vi "Kto_był_pierwszy_SUBVI.vi"(6 "Brama 2":T2, 7 "Brama 1":T2, 9 "Wejscie":T1) -> (3 "output cluster":T1)   [LabVIEW 2017]
panel:
  in  "Cluster":T1
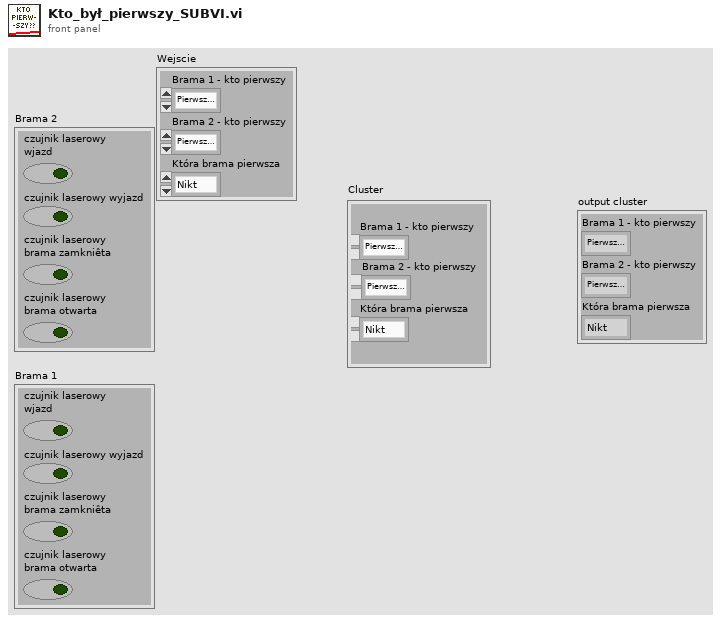
[diagram p1: front panel]
types:
  T1 = cluster{"Brama 1 - kto pierwszy":enum16{"Pierwszy wjazd", "Nikt", "Pierwszy wyjazd"}, "Brama 2 - kto pierwszy":enum16{"Pierwszy wjazd", "Nikt", "Pierwszy wyjazd"}, "Która brama pierwsza":enum16{"Nikt", "Brama 1", "Brama 2"}}
  T2 = cluster{"czujnik laserowy \nwjazd":bool, "czujnik laserowy wyjazd":bool, "czujnik laserowy \nbrama zamkniêta":bool, "czujnik laserowy \nbrama otwarta":bool}
  T3 = enum16{"Pierwszy wjazd", "Nikt", "Pierwszy wyjazd"}
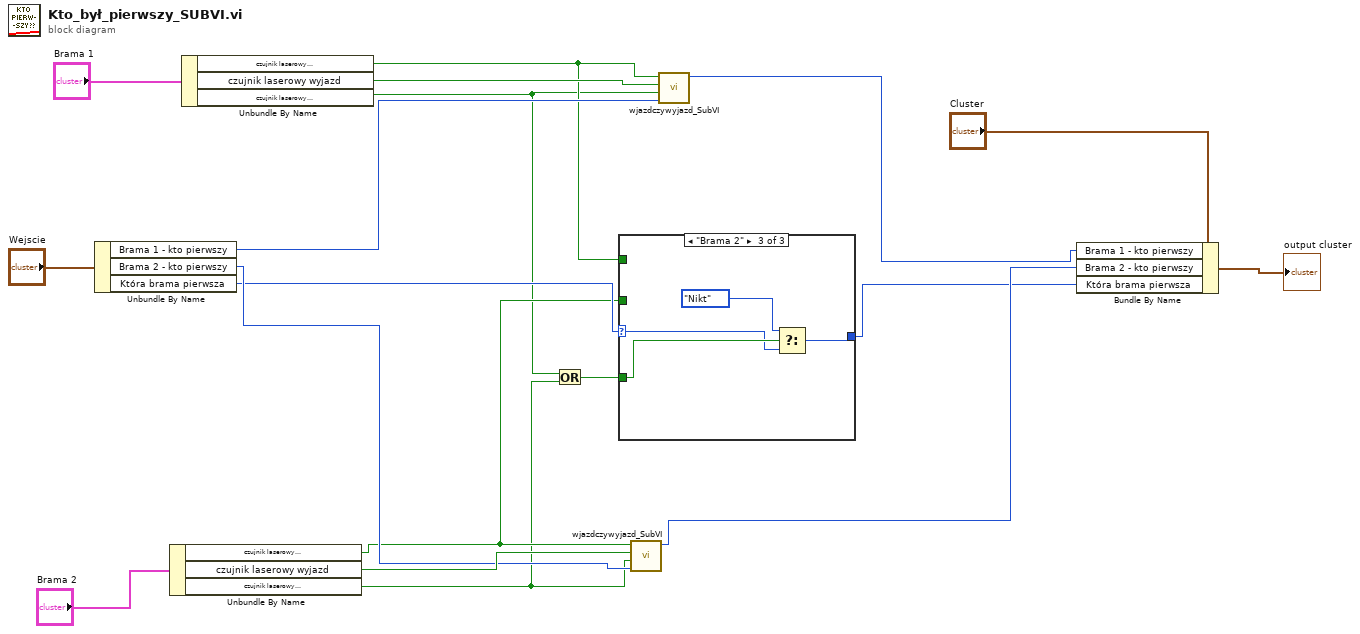
[diagram p0: block diagram]
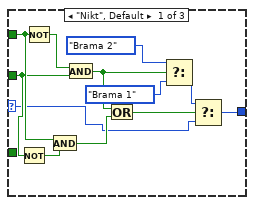
[diagram p2: hidden frame]
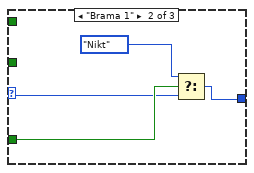
[diagram p3: hidden frame]
diagram:
  n1 = Unbundle By Name("Wejscie") -> ("Brama 1 - kto pierwszy"=w9:T3, "Brama 2 - kto pierwszy"=w8:T3, "Która brama pierwsza"=w7:enum16{"Nikt", "Brama 1", "Brama 2"})
  n2 = Unbundle By Name("Brama 2") -> ("czujnik laserowy \nwjazd"=w5:bool, "czujnik laserowy wyjazd"=w15:bool, "czujnik laserowy \nbrama otwarta"=w3:bool)
  n3 = Unbundle By Name("Brama 1") -> ("czujnik laserowy \nwjazd"=w6:bool, "czujnik laserowy wyjazd"=w16:bool, "czujnik laserowy \nbrama otwarta"=w2:bool)
  n4 = Or(x=w2, y=w3) -> (x .or. y?=w1:bool)
  n5 = case shown="\"Brama 2\"" w7 {
    selector: w7 -> [w24 w32 w36]
    tunnel: w6 -> [w29 _ _]
    tunnel: w5 -> [w28 _ _]
    tunnel: [w19 w31 w38] -> w4
    tunnel: w1 -> [_ w34 w37]
    frame "Nikt", Default {
      n6 = Not(x=w28) -> (.not. x?=w27:bool)
      n7 = Not(x=w29) -> (.not. x?=w30:bool)
      n8 = And(x=w29, y=w27) -> (x .and. y?=w26:bool)
      n9 = And(x=w30, y=w28) -> (x .and. y?=w22:bool)
      n10 = Or(x=w22, y=w26) -> (x .or. y?=w25:bool)
      n11 = Select(t=enum16{"Nikt", "Brama 1", "Brama 2"}."Brama 2", s=w22, f=enum16{"Nikt", "Brama 1", "Brama 2"}."Brama 1") -> (s? t:f=w23:enum16{"Nikt", "Brama 1", "Brama 2"})
      n12 = Select(t=w23, s=w25, f=w24) -> (s? t:f=w19:enum16{"Nikt", "Brama 1", "Brama 2"})
    }
    frame "Brama 1" {
      n13 = Select(t=enum16{"Nikt", "Brama 1", "Brama 2"}."Nikt", s=w34, f=w32) -> (s? t:f=w31:enum16{"Nikt", "Brama 1", "Brama 2"})
    }
    frame "Brama 2" {
      n14 = Select(t=enum16{"Nikt", "Brama 1", "Brama 2"}."Nikt", s=w37, f=w36) -> (s? t:f=w38:enum16{"Nikt", "Brama 1", "Brama 2"})
    }
  }
  n15 = call "wjazdczywyjazd_SubVI.vi"("WE"=w8, "czujnik laserowy \nbrama otwarta"=w3, "czujnik laserowy wyjazd"=w15, "czujnik laserowy \nwjazd"=w5) -> ("Enum"=w12:T3)  [unwired: 7 in]
  n16 = call "wjazdczywyjazd_SubVI.vi"("WE"=w9, "czujnik laserowy \nbrama otwarta"=w2, "czujnik laserowy wyjazd"=w16, "czujnik laserowy \nwjazd"=w6) -> ("Enum"=w13:T3)  [unwired: 7 in]
  n17 = Bundle By Name(cluster="Cluster", "Brama 1 - kto pierwszy"=w13, "Brama 2 - kto pierwszy"=w12, "Która brama pierwsza"=w4) -> (→"output cluster":T1)
